vi "Write ContinueEventRate [ms].vi"(8 "error in (no error)":errorcluster, 10 "ContinueEventRate [ms]":u32=100, 11 "ActorStateMachine in":refnum<class "ActorStateMachine.lvclass">) -> (0 "error out":errorcluster, 3 "ActorStateMachine out":refnum<class "ActorStateMachine.lvclass">)   [LabVIEW 2021, in "ActorStateMachine.lvlib" / "ActorStateMachine.lvclass"]
uses:
  ActorStateMachine.lvclass
  ActorStateMachine.lvclass/ActorStateMachine.ctl
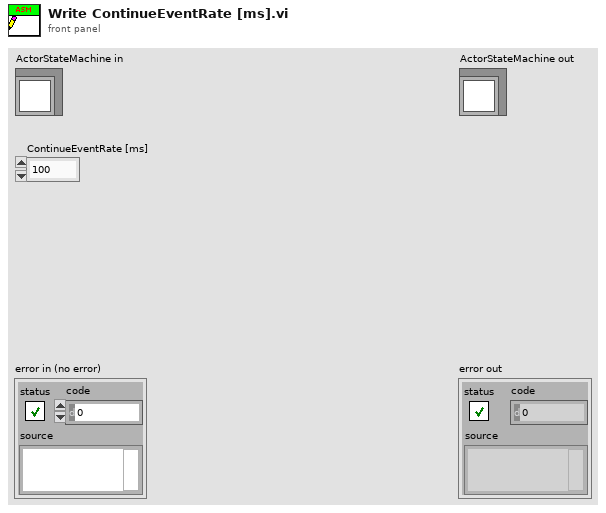
[diagram p1: front panel]
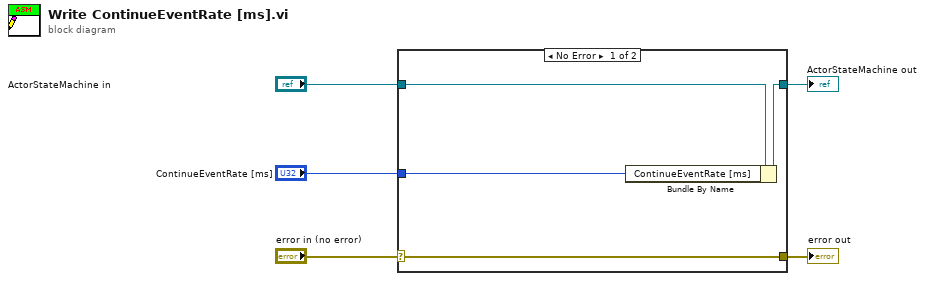
[diagram p0: block diagram]
diagram:
  n1 = case shown="No Error" "error in (no error)" {
    selector: "error in (no error)" -> [w9 w10]
    tunnel: [w9 w10] -> w4
    tunnel: [w7 w11] -> w2
    tunnel: "ActorStateMachine in" -> [w8 w11]
    tunnel: "ContinueEventRate [ms]" -> [w6 _]
    frame No Error {
      n2 = Bundle By Name(cluster=w8, "ContinueEventRate [ms]"=w6) -> (w7:refnum<class "ActorStateMachine.lvclass">)
    }
    frame Error {
    }
  }
  "error out" <- w4
  "ActorStateMachine out" <- w2
